vi "To Waveform.vi"(8 "error in (no error)":errorcluster, 11 "Boolean Array in":refnum<class "Boolean Array.lvclass">) -> (0 "error out":errorcluster, 1 "Success?":bool, 3 "Waveform Array":waveform(dbl)[](array[waveform]))   [LabVIEW 2020, in "Data.lvlib" / "Boolean Array.lvclass"]
doc: "Interpret 'Data' as a Waveform Array. If impossible 'Success?' is set to FALSE"
uses:
  Boolean Array.lvclass
  Boolean Array.lvclass/Boolean Array.ctl
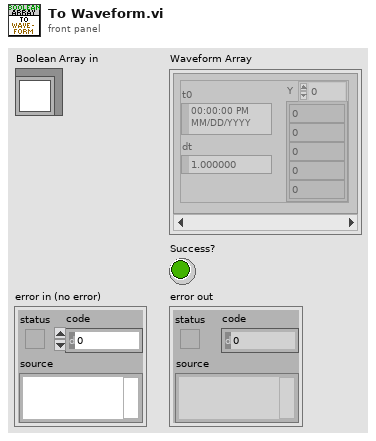
[diagram p1: front panel]
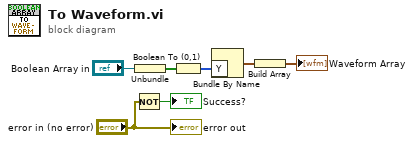
[diagram p0: block diagram]
diagram:
  n1 = Not(x="error in (no error)") -> (.not. x?=→"Success?":bool)
  n2 = Unbundle("Boolean Array in") -> (w6:bool[])
  n3 = Boolean To (0,1)(Boolean=w6) -> (0, 1=w5:i16[])
  n4 = Bundle By Name("Y"=w5) -> (w4:waveform(i16))  [unwired: 1 in]
  n5 = Build Array(w4) -> (→"Waveform Array":waveform(i16)[])
  "error out" <- "error in (no error)"
